vi "Parameter_szamolas.vi"(8 "Tbelsolevego_0":dbl=20.5 format="%#_13g", 9 "Bemeneti paraméterek":T2={"rho PCM"=1100.0, "rho kulso"=28.3, "Dkulso"=0.1, "nkulso"=10, "rho kozepso"=28.3, "Dkozepso"=0.06, "nkozepso"=6, "rho belso"=28.3, "Dbelso"=0.1, "nbelso"=10, "Alfa kulso"=0.015, "Alfa belso"=0.006, "Alfa kont"=0.03, "lambda_kulso"=5.0000000000105516e-05, "lambda_kozepso"=5e-05, "lambda_belso"=5e-05, "hpcm_olv"=140.0, "Top_also"=24.0, "Top_felso"=28.0, "ckulso"=1.13, "ckozepso"=1.13, "cbelso"=1.13, "cpcm_szilard"=1.9, "lambda_pcm"=0.00018, "Vlevego"=0.446, "rho levego"=1.3, "clevego"=1.0, "cpcm_olvnelkul"=0.0, "cpcm_foly"=1.5, "Xpcm_kulso"=0.3, "Xpcm_belso"=0.3}, 10 "Parameterek":T3={"rholevego"=1.3, "Vlevego"=0.446, "Mlevego"=0.0, "clevego"=1.0, "rho PCM"=1100.0, "rho kulso"=28.3, "Dkulso"=0.1, "nkulso"=10, "dkulso"=0.0, "vkulso"=0.0, "rho kozepso"=28.3, "Dkozepso"=0.06, "nkozepso"=6, "dkozepso"=0.0, "vkozepso"=0.0, "mkozepso"=0.0, "mkulso"=0.0, "rho belso"=28.3, "Dbelso"=0.1, "nbelso"=10, "dbelso"=0.0, "vbelso"=0.0, "mbelso"=0.0, "Xpcm_kulso"=0.3, "Xpcm_belso"=0.3, "mpcm_kulso"=0.0, "mpcm_belso"=0.0, "mkulso_pcm"=0.0, "mbelso_pcm"=0.0, "ckulso"=1.13, "ckozepso"=1.13, "cbelso"=1.13, "cpcm_szilard"=1.9, "cpcm_foly"=1.5, "ckulso_Topalatt"=0.0, "cbelso_Topalatt"=0.0, "ckulso_Topfelett"=0.0, "cbelso_Topfelett"=0.0, "hpcm_olv"=140.0, "ckulso_eff_Tolv"=0.0, "cbelso_eff_Tolv"=0.0, "Qkulso_op_also"=0.0, "Qkulso_op_felso"=0.0, "Qbelso_op_also"=0.0, "Qbelso_op_felso"=0.0, "lambda_kulso"=5e-05, "lambda_kozepso"=5e-05, "lambda_belso"=5e-05, "lambda_pcm"=0.00018, "VXpcm_kulso"=0.0, "VXpcm_belso"=0.0, "lambda_kulsoPCM"=0.0, "lambda_belsoPCM"=0.0, "Alfa_kulso"=0.015, "Alfa_belso"=0.006, "Alfa_kont"=0.03, "Top_also"=24.0, "Top_felso"=28.0, "cpcm_olvnelkul"=1.0, "Tbelsolevego_0"=22.0}) -> (1 "Számolt paraméterek":T1, 2 "Parameterek 2":T3={"rholevego"=0.0, "Vlevego"=0.0, "Mlevego"=0.0, "clevego"=0.0, "rho PCM"=1100.0, "rho kulso"=28.3, "Dkulso"=0.1, "nkulso"=10, "dkulso"=0.0, "vkulso"=0.0, "rho kozepso"=28.3, "Dkozepso"=0.06, "nkozepso"=6, "dkozepso"=0.0, "vkozepso"=0.0, "mkozepso"=0.0, "mkulso"=0.0, "rho belso"=28.3, "Dbelso"=0.1, "nbelso"=10, "dbelso"=0.0, "vbelso"=0.0, "mbelso"=0.0, "Xpcm_kulso"=0.3, "Xpcm_belso"=0.3, "mpcm_kulso"=0.0, "mpcm_belso"=0.0, "mkulso_pcm"=0.0, "mbelso_pcm"=0.0, "ckulso"=1.13, "ckozepso"=1.13, "cbelso"=1.13, "cpcm_szilard"=1.9, "cpcm_foly"=1.5, "ckulso_Topalatt"=0.0, "cbelso_Topalatt"=0.0, "ckulso_Topfelett"=0.0, "cbelso_Topfelett"=0.0, "hpcm_olv"=140.0, "ckulso_eff_Tolv"=0.0, "cbelso_eff_Tolv"=0.0, "Qkulso_op_also"=0.0, "Qkulso_op_felso"=0.0, "Qbelso_op_also"=0.0, "Qbelso_op_felso"=0.0, "lambda_kulso"=5e-05, "lambda_kozepso"=5e-05, "lambda_belso"=5e-05, "lambda_pcm"=0.00018, "VXpcm_kulso"=0.0, "VXpcm_belso"=0.0, "lambda_kulsoPCM"=0.0, "lambda_belsoPCM"=0.0, "Alfa_kulso"=0.015, "Alfa_belso"=0.006, "Alfa_kont"=0.03, "Top_also"=24.0, "Top_felso"=28.0, "cpcm_olvnelkul"=0.0, "Tbelsolevego_0"=22.0})   [LabVIEW 2013]
uses:
  Parameterek.ctl
  Bemeno_Parameterek.ctl
  Szamolt_Parameterek.ctl
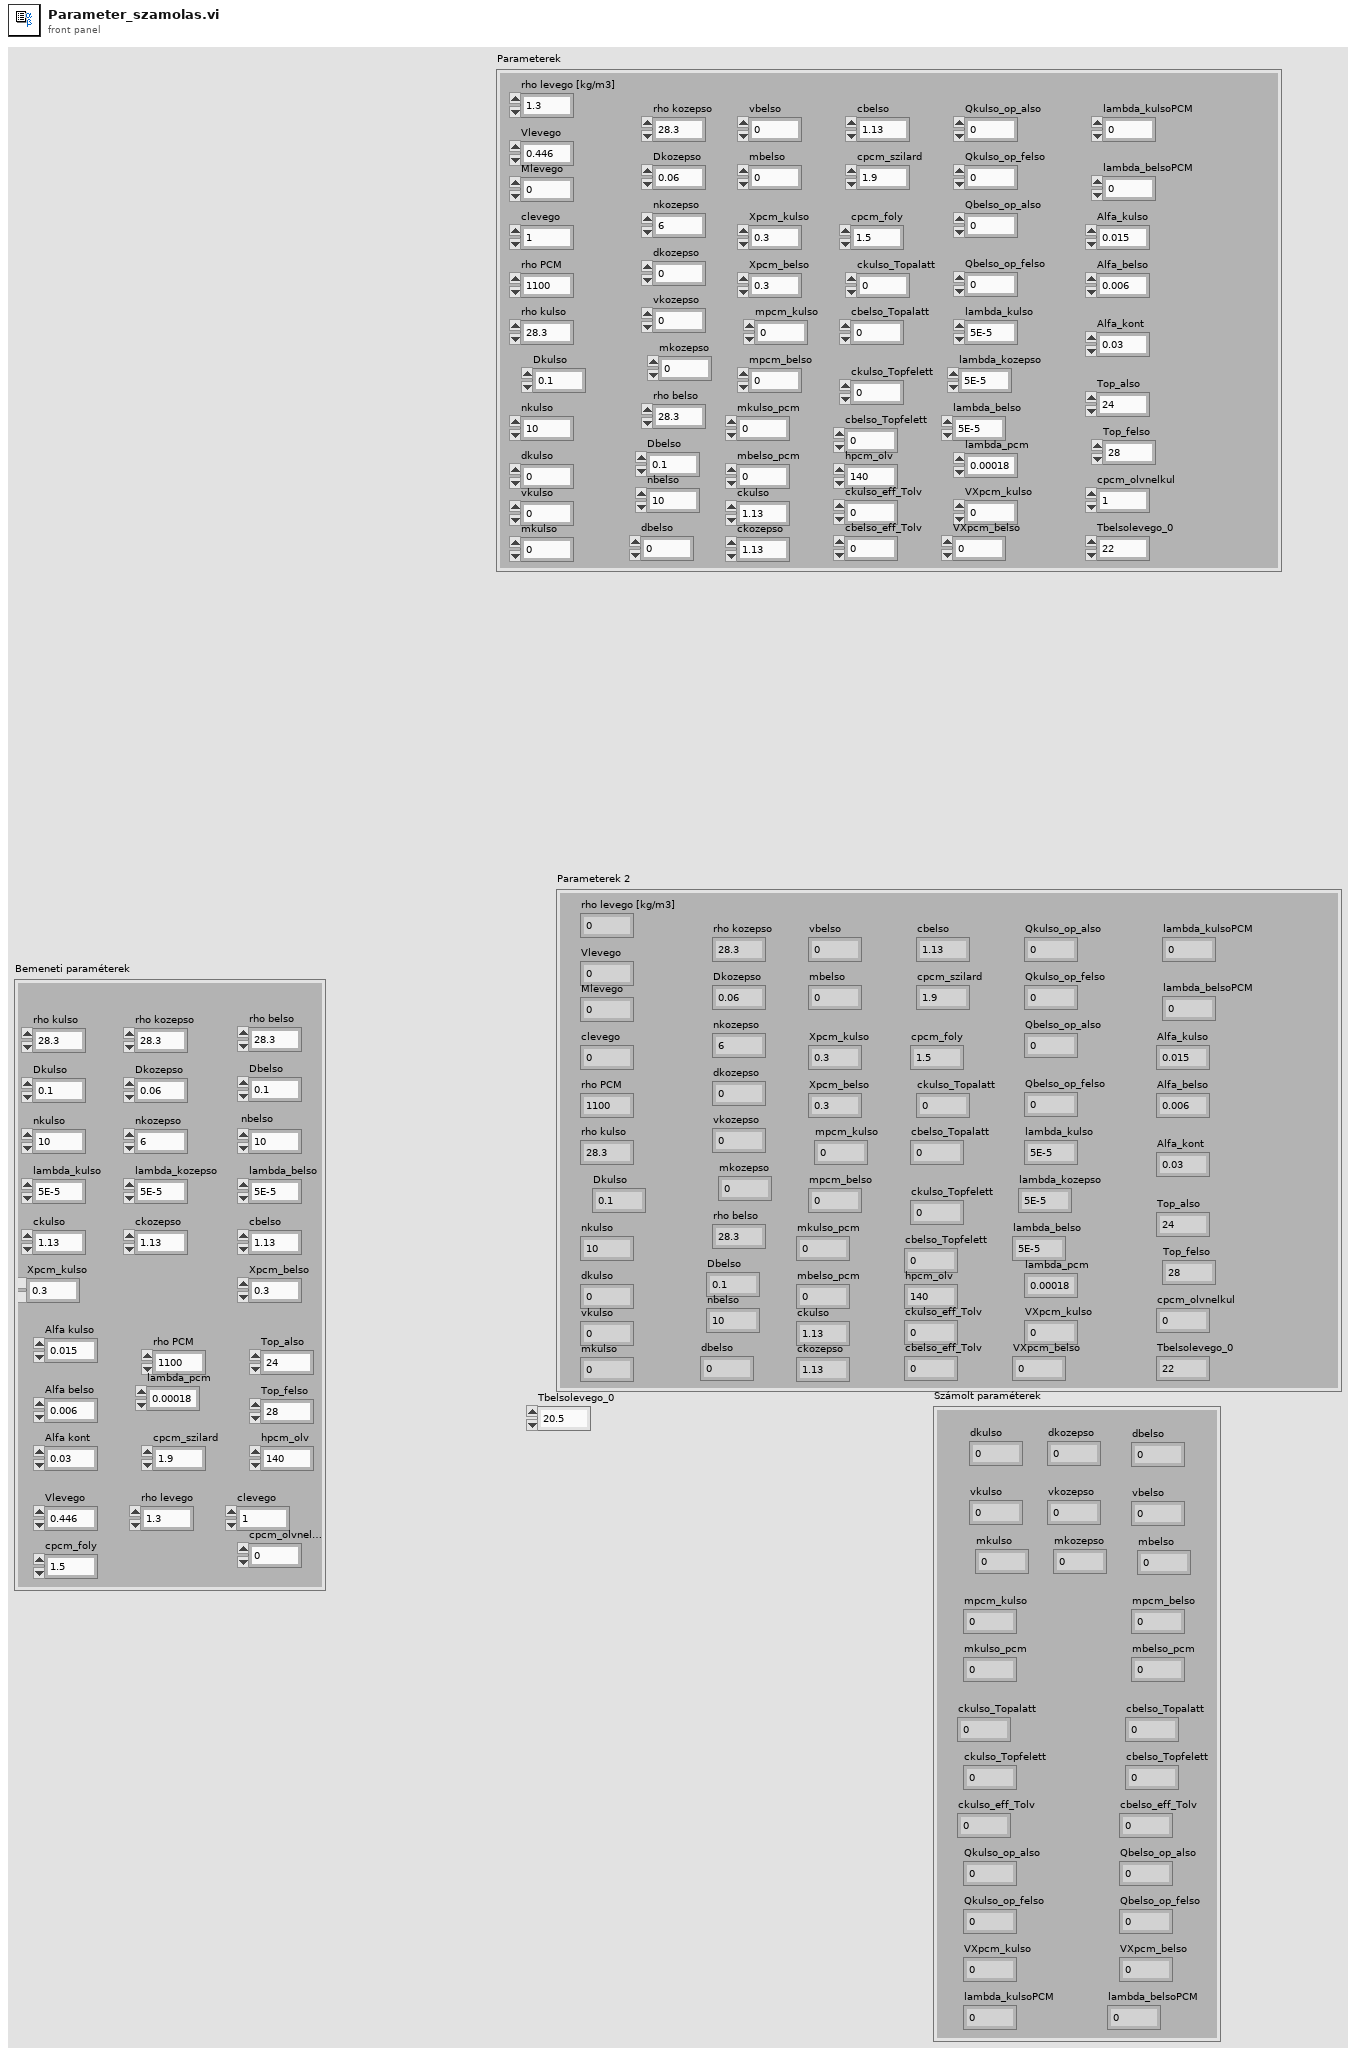
[diagram p1: front panel]
types:
  T1 = typedef "Szamolt_Parameterek.ctl" = cluster{"dkulso":dbl, "dkozepso":dbl, "dbelso":dbl, "vkulso":dbl, "vkozepso":dbl, "vbelso":dbl, "mkulso":dbl, "mkozepso":dbl, "mbelso":dbl, "mpcm_kulso":dbl, "mpcm_belso":dbl, "mkulso_pcm":dbl, "mbelso_pcm":dbl, "ckulso_Topalatt":dbl, "ckulso_Topfelett":dbl, "cbelso_Topalatt":dbl, "cbelso_Topfelett":dbl, "ckulso_eff_Tolv":dbl, "cbelso_eff_Tolv":dbl, "Qkulso_op_also":dbl, "Qkulso_op_felso":dbl, "Qbelso_op_also":dbl, "Qbelso_op_felso":dbl, "VXpcm_kulso":dbl, "VXpcm_belso":dbl, "lambda_kulsoPCM":dbl, "lambda_belsoPCM":dbl}
  T2 = typedef "Bemeno_Parameterek.ctl" = cluster{"rho PCM":dbl, "rho kulso":dbl, "Dkulso":dbl, "nkulso":i32, "rho kozepso":dbl, "Dkozepso":dbl, "nkozepso":i32, "rho belso":dbl, "Dbelso":dbl, "nbelso":i32, "Alfa kulso":dbl, "Alfa belso":dbl, "Alfa kont":dbl, "lambda_kulso":dbl, "lambda_kozepso":dbl, "lambda_belso":dbl, "hpcm_olv":dbl, "Top_also":dbl, "Top_felso":dbl, "ckulso":dbl, "ckozepso":dbl, "cbelso":dbl, "cpcm_szilard":dbl, "lambda_pcm":dbl, "Vlevego":dbl, "rho levego":dbl, "clevego":dbl, "cpcm_olvnelkul":dbl, "cpcm_foly":dbl, "Xpcm_kulso":dbl, "Xpcm_belso":dbl}
  T3 = typedef "Parameterek.ctl" = cluster{"rholevego":dbl, "Vlevego":dbl, "Mlevego":dbl, "clevego":dbl, "rho PCM":dbl, "rho kulso":dbl, "Dkulso":dbl, "nkulso":i32, "dkulso":dbl, "vkulso":dbl, "rho kozepso":dbl, "Dkozepso":dbl, "nkozepso":i32, "dkozepso":dbl, "vkozepso":dbl, "mkozepso":dbl, "mkulso":dbl, "rho belso":dbl, "Dbelso":dbl, "nbelso":i32, "dbelso":dbl, "vbelso":dbl, "mbelso":dbl, "Xpcm_kulso":dbl, "Xpcm_belso":dbl, "mpcm_kulso":dbl, "mpcm_belso":dbl, "mkulso_pcm":dbl, "mbelso_pcm":dbl, "ckulso":dbl, "ckozepso":dbl, "cbelso":dbl, "cpcm_szilard":dbl, "cpcm_foly":dbl, "ckulso_Topalatt":dbl, "cbelso_Topalatt":dbl, "ckulso_Topfelett":dbl, "cbelso_Topfelett":dbl, "hpcm_olv":dbl, "ckulso_eff_Tolv":dbl, "cbelso_eff_Tolv":dbl, "Qkulso_op_also":dbl, "Qkulso_op_felso":dbl, "Qbelso_op_also":dbl, "Qbelso_op_felso":dbl, "lambda_kulso":dbl, "lambda_kozepso":dbl, "lambda_belso":dbl, "lambda_pcm":dbl, "VXpcm_kulso":dbl, "VXpcm_belso":dbl, "lambda_kulsoPCM":dbl, "lambda_belsoPCM":dbl, "Alfa_kulso":dbl, "Alfa_belso":dbl, "Alfa_kont":dbl, "Top_also":dbl, "Top_felso":dbl, "cpcm_olvnelkul":dbl, "Tbelsolevego_0":dbl}
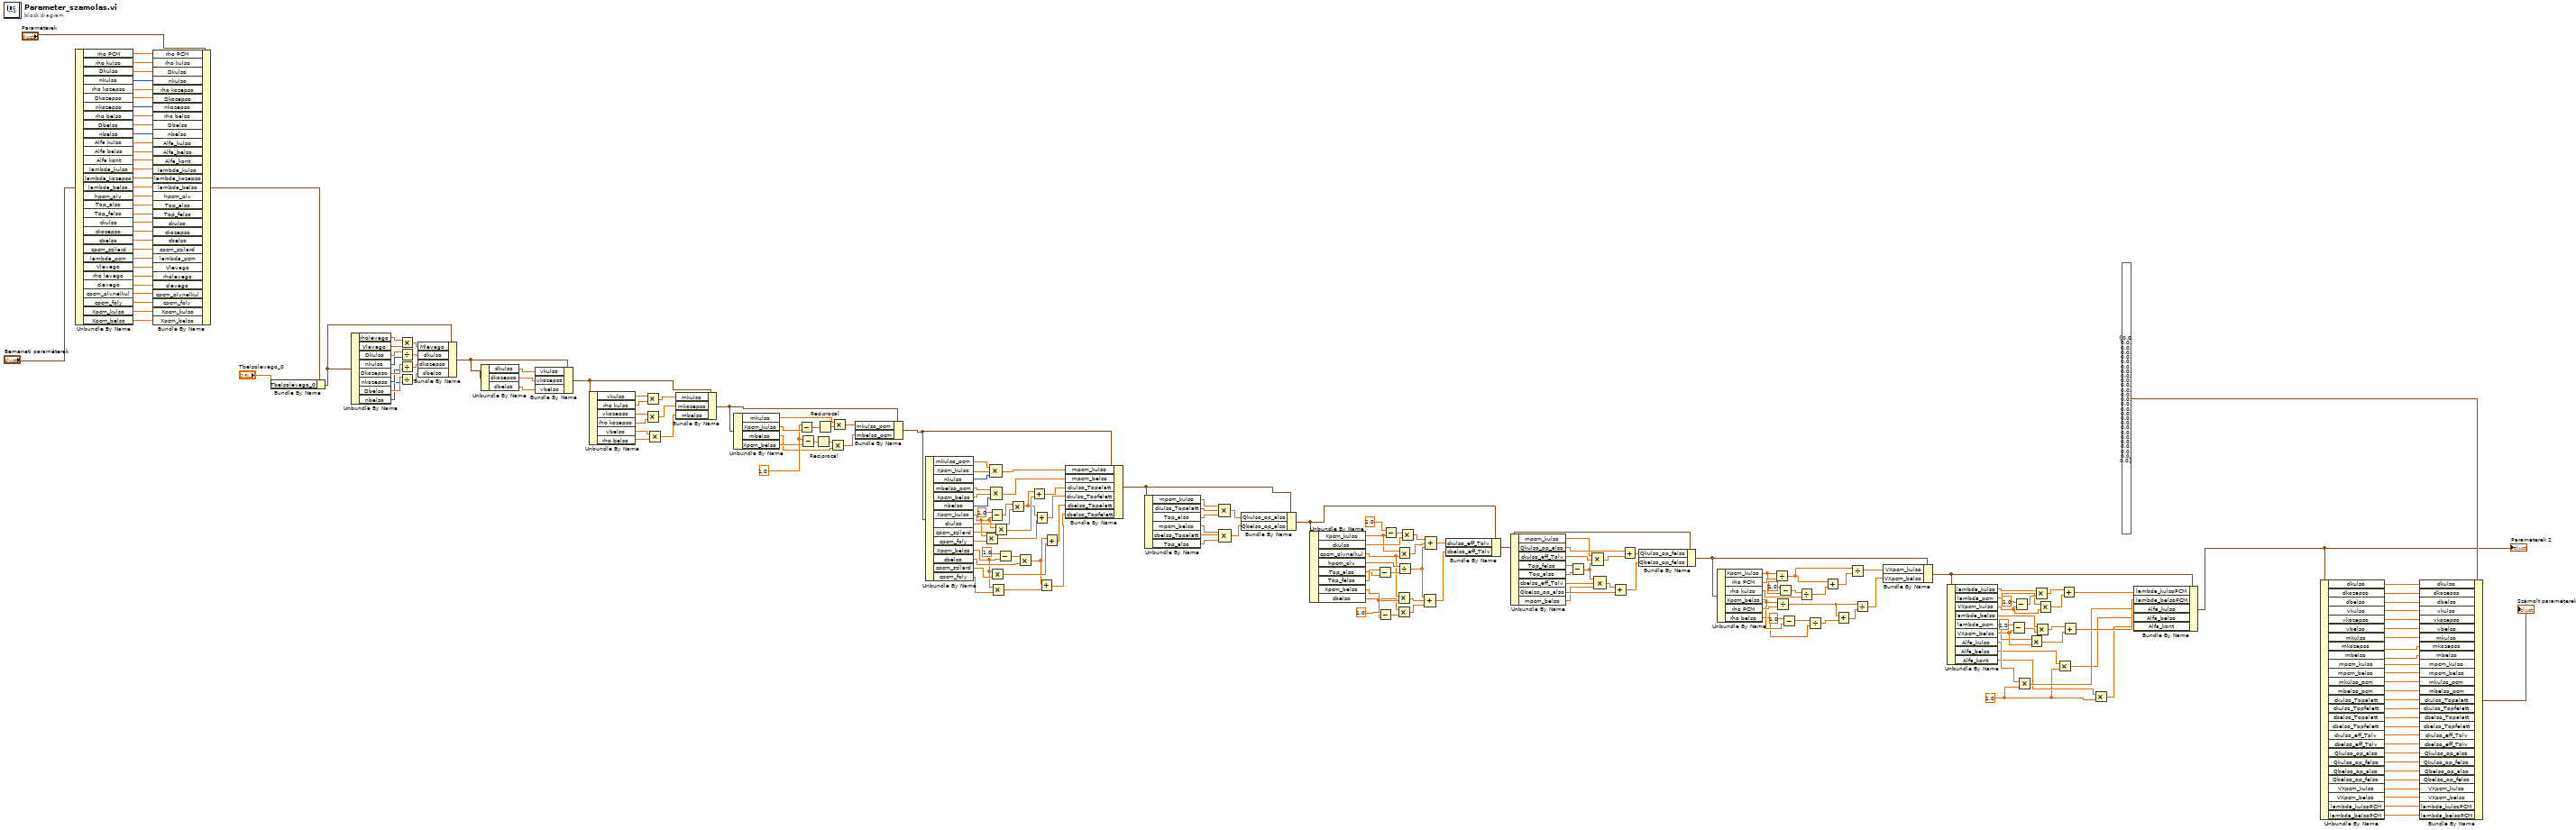
[diagram p0: block diagram]
diagram:
  w73 = 1.0 ("y")
  w188 = 1.0
  n1 = Unbundle By Name("Bemeneti paraméterek") -> ("rho PCM"=w61:dbl, "rho kulso"=w58:dbl, "Dkulso"=w59:dbl, "nkulso"=w60:i32, "rho kozepso"=w57:dbl, "Dkozepso"=w56:dbl, "nkozepso"=w55:i32, "rho belso"=w54:dbl, "Dbelso"=w53:dbl, "nbelso"=w52:i32, "Alfa kulso"=w51:dbl, "Alfa belso"=w50:dbl, "Alfa kont"=w49:dbl, "lambda_kulso"=w48:dbl, "lambda_kozepso"=w47:dbl, "lambda_belso"=w46:dbl, "hpcm_olv"=w45:dbl, "Top_also"=w44:dbl, "Top_felso"=w43:dbl, "ckulso"=w42:dbl, "ckozepso"=w41:dbl, "cbelso"=w40:dbl, "cpcm_szilard"=w39:dbl, "lambda_pcm"=w38:dbl, "Vlevego"=w37:dbl, "rho levego"=w36:dbl, "clevego"=w35:dbl, "cpcm_olvnelkul"=w34:dbl, "cpcm_foly"=w33:dbl, "Xpcm_kulso"=w32:dbl, "Xpcm_belso"=w31:dbl)
  n2 = Bundle By Name(cluster="Parameterek", "rho PCM"=w61, "rho kulso"=w58, "Dkulso"=w59, "nkulso"=w60, "rho kozepso"=w57, "Dkozepso"=w56, "nkozepso"=w55, "rho belso"=w54, "Dbelso"=w53, "nbelso"=w52, "Alfa_kulso"=w51, "Alfa_belso"=w50, "Alfa_kont"=w49, "lambda_kulso"=w48, "lambda_kozepso"=w47, "lambda_belso"=w46, "hpcm_olv"=w45, "Top_also"=w44, "Top_felso"=w43, "ckulso"=w42, "ckozepso"=w41, "cbelso"=w40, "cpcm_szilard"=w39, "lambda_pcm"=w38, "Vlevego"=w37, "rholevego"=w36, "clevego"=w35, "cpcm_olvnelkul"=w34, "cpcm_foly"=w33, "Xpcm_kulso"=w32, "Xpcm_belso"=w31) -> (w63:T3)
  n3 = Bundle By Name(cluster=w63, "Tbelsolevego_0"="Tbelsolevego_0") -> (w80:T3)
  n4 = Unbundle By Name(w80) -> ("rholevego"=w222:dbl, "Vlevego"=w221:dbl, "Dkulso"=w219:dbl, "nkulso"=w218:i32, "Dkozepso"=w216:dbl, "nkozepso"=w215:i32, "Dbelso"=w213:dbl, "nbelso"=w212:i32)
  n5 = Multiply(x=w222, y=w221) -> (x*y=w220:dbl)
  n6 = Divide(x=w219, y=w218) -> (x/y=w217:dbl)
  n7 = Divide(x=w216, y=w215) -> (x/y=w214:dbl)
  n8 = Divide(x=w213, y=w212) -> (x/y=w211:dbl)
  n9 = Bundle By Name(cluster=w80, "Mlevego"=w220, "dkulso"=w217, "dkozepso"=w214, "dbelso"=w211) -> (w210:T3)
  n10 = Unbundle By Name(w210) -> ("dkulso"=w209:dbl, "dkozepso"=w208:dbl, "dbelso"=w207:dbl)
  n11 = Bundle By Name(cluster=w210, "vkulso"=w209, "vkozepso"=w208, "vbelso"=w207) -> (w206:T3)
  n12 = Unbundle By Name(w206) -> ("vkulso"=w205:dbl, "rho kulso"=w204:dbl, "vkozepso"=w200:dbl, "rho kozepso"=w199:dbl, "vbelso"=w198:dbl, "rho belso"=w197:dbl)
  n13 = Multiply(x=w205, y=w204) -> (x*y=w203:dbl)
  n14 = Multiply(x=w200, y=w199) -> (x*y=w202:dbl)
  n15 = Multiply(x=w198, y=w197) -> (x*y=w201:dbl)
  n16 = Bundle By Name(cluster=w206, "mkulso"=w203, "mkozepso"=w202, "mbelso"=w201) -> (w196:T3)
  n17 = Unbundle By Name(w196) -> ("mkulso"=w193:dbl, "Xpcm_kulso"=w195:dbl, "mbelso"=w186:dbl, "Xpcm_belso"=w187:dbl)
  n18 = Subtract(x=w188, y=w195) -> (x-y=w191:dbl)
  n19 = Subtract(x=w188, y=w187) -> (x-y=w190:dbl)
  n20 = Reciprocal(x=w190) -> (1/x=w189:dbl)
  n21 = Reciprocal(x=w191) -> (1/x=w194:dbl)
  n22 = Multiply(x=w189, y=w186) -> (x*y=w185:dbl)
  n23 = Multiply(x=w193, y=w194) -> (x*y=w192:dbl)
  n24 = Bundle By Name(cluster=w196, "mkulso_pcm"=w192, "mbelso_pcm"=w185) -> (w183:T3)
  n25 = Unbundle By Name(w183) -> ("mkulso_pcm"=w182:dbl, "Xpcm_kulso"=w181:dbl, "nkulso"=w180:i32, "mbelso_pcm"=w179:dbl, "Xpcm_belso"=w178:dbl, "nbelso"=w177:i32, "Xpcm_kulso"=w168:dbl, "ckulso"=w173:dbl, "cpcm_szilard"=w172:dbl, "cpcm_foly"=w169:dbl, "Xpcm_belso"=w157:dbl, "cbelso"=w162:dbl, "cpcm_szilard"=w161:dbl, "cpcm_foly"=w158:dbl)
  n26 = Multiply(x=w168, y=w169) -> (x*y=w167:dbl)
  n27 = Subtract(x=1.0, y=w168) -> (x-y=w174:dbl)
  n28 = Multiply(x=w157, y=w161) -> (x*y=w160:dbl)
  n29 = Compound Arithmetic op=MULTIPLY(w182, w181, w180) -> (w184:dbl)
  n30 = Multiply(x=w157, y=w158) -> (x*y=w156:dbl)
  n31 = Compound Arithmetic op=MULTIPLY(w179, w178, w177) -> (w176:dbl)
  n32 = Multiply(x=w168, y=w172) -> (x*y=w171:dbl)
  n33 = Subtract(x=1.0, y=w157) -> (x-y=w163:dbl)
  n34 = Multiply(x=w174, y=w173) -> (x*y=w166:dbl)
  n35 = Multiply(x=w163, y=w162) -> (x*y=w155:dbl)
  n36 = Add(x=w166, y=w171) -> (x+y=w170:dbl)
  n37 = Add(x=w166, y=w167) -> (x+y=w165:dbl)
  n38 = Add(x=w155, y=w156) -> (x+y=w154:dbl)
  n39 = Add(x=w155, y=w160) -> (x+y=w159:dbl)
  n40 = Bundle By Name(cluster=w183, "mpcm_kulso"=w184, "mpcm_belso"=w176, "ckulso_Topalatt"=w170, "ckulso_Topfelett"=w165, "cbelso_Topalatt"=w159, "cbelso_Topfelett"=w154) -> (w153:T3)
  n41 = Unbundle By Name(w153) -> ("mpcm_kulso"=w152:dbl, "ckulso_Topalatt"=w151:dbl, "Top_also"=w150:dbl, "mpcm_belso"=w148:dbl, "cbelso_Topalatt"=w147:dbl, "Top_also"=w146:dbl)
  n42 = Compound Arithmetic op=MULTIPLY(w152, w151, w150) -> (w149:dbl)
  n43 = Compound Arithmetic op=MULTIPLY(w148, w147, w146) -> (w145:dbl)
  n44 = Bundle By Name(cluster=w153, "Qkulso_op_also"=w149, "Qbelso_op_also"=w145) -> (w144:T3)
  n45 = Unbundle By Name(w144) -> ("Xpcm_kulso"=w139:dbl, "ckulso"=w141:dbl, "cpcm_olvnelkul"=w132:dbl, "hpcm_olv"=w135:dbl, "Top_also"=w136:dbl, "Top_felso"=w137:dbl, "Xpcm_belso"=w128:dbl, "cbelso"=w126:dbl)
  n46 = Subtract(x=w137, y=w136) -> (x-y=w134:dbl)
  n47 = Subtract(x=1.0, y=w128) -> (x-y=w127:dbl)
  n48 = Subtract(x=1.0, y=w139) -> (x-y=w142:dbl)
  n49 = Multiply(x=w132, y=w128) -> (x*y=w131:dbl)
  n50 = Multiply(x=w126, y=w127) -> (x*y=w125:dbl)
  n51 = Multiply(x=w139, y=w132) -> (x*y=w138:dbl)
  n52 = Divide(x=w135, y=w134) -> (x/y=w130:dbl)
  n53 = Multiply(x=w142, y=w141) -> (x*y=w140:dbl)
  n54 = Compound Arithmetic op=ADD(w130, w131, w125) -> (w124:dbl)
  n55 = Compound Arithmetic op=ADD(w140, w138, w130) -> (w133:dbl)
  n56 = Bundle By Name(cluster=w144, "ckulso_eff_Tolv"=w133, "cbelso_eff_Tolv"=w124) -> (w123:T3)
  n57 = Unbundle By Name(w123) -> ("mpcm_kulso"=w70:dbl, "Qkulso_op_also"=w121:dbl, "ckulso_eff_Tolv"=w71:dbl, "Top_felso"=w120:dbl, "Top_also"=w119:dbl, "cbelso_eff_Tolv"=w67:dbl, "Qbelso_op_also"=w118:dbl, "mpcm_belso"=w66:dbl)
  n58 = Subtract(x=w120, y=w119) -> (x-y=w68:dbl)
  n59 = Compound Arithmetic op=MULTIPLY(w70, w71, w68) -> (w69:dbl)
  n60 = Compound Arithmetic op=MULTIPLY(w68, w67, w66) -> (w65:dbl)
  n61 = Add(x=w65, y=w118) -> (x+y=w117:dbl)
  n62 = Add(x=w121, y=w69) -> (x+y=w122:dbl)
  n63 = Bundle By Name(cluster=w123, "Qkulso_op_felso"=w122, "Qbelso_op_felso"=w117) -> (w116:T3)
  n64 = Unbundle By Name(w116) -> ("Xpcm_kulso"=w111:dbl, "rho PCM"=w115:dbl, "rho kulso"=w109:dbl, "Xpcm_belso"=w103:dbl, "rho PCM"=w105:dbl, "rho belso"=w98:dbl)
  n65 = Divide(x=w111, y=w115) -> (x/y=w113:dbl)
  n66 = Divide(x=w103, y=w105) -> (x/y=w101:dbl)
  n67 = Subtract(x=1.0, y=w111) -> (x-y=w110:dbl)
  n68 = Subtract(x=1.0, y=w103) -> (x-y=w99:dbl)
  n69 = Divide(x=w110, y=w109) -> (x/y=w108:dbl)
  n70 = Divide(x=w99, y=w98) -> (x/y=w100:dbl)
  n71 = Add(x=w113, y=w108) -> (x+y=w107:dbl)
  n72 = Add(x=w101, y=w100) -> (x+y=w102:dbl)
  n73 = Divide(x=w113, y=w107) -> (x/y=w114:dbl)
  n74 = Divide(x=w101, y=w102) -> (x/y=w106:dbl)
  n75 = Bundle By Name(cluster=w116, "VXpcm_kulso"=w114, "VXpcm_belso"=w106) -> (w97:T3)
  n76 = Unbundle By Name(w97) -> ("lambda_kulso"=w94:dbl, "lambda_pcm"=w89:dbl, "VXpcm_kulso"=w90:dbl, "lambda_belso"=w84:dbl, "lambda_pcm"=w83:dbl, "VXpcm_belso"=w86:dbl, "Alfa_kulso"=w79:dbl, "Alfa_belso"=w77:dbl, "Alfa_kont"=w75:dbl)
  n77 = Subtract(x=1.0, y=w86) -> (x-y=w85:dbl)
  n78 = Subtract(x=1.0, y=w90) -> (x-y=w95:dbl)
  n79 = Multiply(x=w79, y=w73) -> (x*y=w78:dbl)
  n80 = Multiply(x=w83, y=w86) -> (x*y=w81:dbl)
  n81 = Multiply(x=w94, y=w95) -> (x*y=w93:dbl)
  n82 = Multiply(x=w84, y=w85) -> (x*y=w82:dbl)
  n83 = Multiply(x=w89, y=w90) -> (x*y=w88:dbl)
  n84 = Multiply(x=w77, y=w73) -> (x*y=w76:dbl)
  n85 = Add(x=w93, y=w88) -> (x+y=w92:dbl)
  n86 = Add(x=w82, y=w81) -> (x+y=w91:dbl)
  n87 = Multiply(x=w75, y=w73) -> (x*y=w74:dbl)
  n88 = Bundle By Name(cluster=w97, "lambda_kulsoPCM"=w92, "lambda_belsoPCM"=w91, "Alfa_kulso"=w78, "Alfa_belso"=w76, "Alfa_kont"=w74) -> (w28:T3)
  "Parameterek 2" <- w28
  n89 = Unbundle By Name(w28) -> ("dkulso"=w27:dbl, "dkozepso"=w26:dbl, "dbelso"=w25:dbl, "vkulso"=w24:dbl, "vkozepso"=w23:dbl, "vbelso"=w22:dbl, "mkulso"=w21:dbl, "mkozepso"=w20:dbl, "mbelso"=w19:dbl, "mpcm_kulso"=w18:dbl, "mpcm_belso"=w17:dbl, "mkulso_pcm"=w16:dbl, "mbelso_pcm"=w15:dbl, "ckulso_Topalatt"=w14:dbl, "ckulso_Topfelett"=w13:dbl, "cbelso_Topalatt"=w12:dbl, "cbelso_Topfelett"=w11:dbl, "ckulso_eff_Tolv"=w10:dbl, "cbelso_eff_Tolv"=w9:dbl, "Qkulso_op_also"=w8:dbl, "Qkulso_op_felso"=w7:dbl, "Qbelso_op_also"=w6:dbl, "Qbelso_op_felso"=w5:dbl, "VXpcm_kulso"=w4:dbl, "VXpcm_belso"=w3:dbl, "lambda_kulsoPCM"=w2:dbl, "lambda_belsoPCM"=w1:dbl)
  n90 = Bundle By Name(cluster=T1 {"dkulso"=0.0, "dkozepso"=0.0, "dbelso"=0.0, "vkulso"=0.0, "vkozepso"=0.0, "vbelso"=0.0, "mkulso"=0.0, "mkozepso"=0.0, "mbelso"=0.0, "mpcm_kulso"=0.0, "mpcm_belso"=0.0, "mkulso_pcm"=0.0, "mbelso_pcm"=0.0, "ckulso_Topalatt"=0.0, "ckulso_Topfelett"=0.0, "cbelso_Topalatt"=0.0, "cbelso_Topfelett"=0.0, "ckulso_eff_Tolv"=0.0, "cbelso_eff_Tolv"=0.0, "Qkulso_op_also"=0.0, "Qkulso_op_felso"=0.0, "Qbelso_op_also"=0.0, "Qbelso_op_felso"=0.0, "VXpcm_kulso"=0.0, "VXpcm_belso"=0.0, "lambda_kulsoPCM"=0.0, "lambda_belsoPCM"=0.0} ("Számolt paraméterek 2"), "dkulso"=w27, "dkozepso"=w26, "dbelso"=w25, "vkulso"=w24, "vkozepso"=w23, "vbelso"=w22, "mkulso"=w21, "mkozepso"=w20, "mbelso"=w19, "mpcm_kulso"=w18, "mpcm_belso"=w17, "mkulso_pcm"=w16, "mbelso_pcm"=w15, "ckulso_Topalatt"=w14, "ckulso_Topfelett"=w13, "cbelso_Topalatt"=w12, "cbelso_Topfelett"=w11, "ckulso_eff_Tolv"=w10, "cbelso_eff_Tolv"=w9, "Qkulso_op_also"=w8, "Qkulso_op_felso"=w7, "Qbelso_op_also"=w6, "Qbelso_op_felso"=w5, "VXpcm_kulso"=w4, "VXpcm_belso"=w3, "lambda_kulsoPCM"=w2, "lambda_belsoPCM"=w1) -> (→"Számolt paraméterek":T1)
